vi "autorampturn.vi"() -> ()   [LabVIEW 2012, in "MainProject.lvrbt"]
uses:
  MainProject.lvrbt
  <vilib>/NXT/Hardware/Plugins/Tetrix DC Motor/TetrixDCMotorAddress.ctl
  Drivers/AutoDriverControl.ctl
  FTC 2012 - 2013/Controls/SpeedControl.ctl
  <vilib>/NXT/HiTechnic/HiTechnic Controls/HiTechnic Port.ctl
  <vilib>/NXT/Block Support/NXT_InputPort.ctl
  <vilib>/NXT/NXTIO Xnodes/NXTIONodeSubVIs/TETRIX IO Check Battery.vi
  <vilib>/NXT/Dual Mode Library/Waits/Wait_Num(msec).vi
  <vilib>/NXT/NXTIO Xnodes/NXTIONodeSubVIs/TETRIX IO Stop DC Motors.vi
  <vilib>/NXT/Subs/LVHSConnector.ctl
  <vilib>/NXT/NXTIO Xnodes/AddressXNode/NXTIOAddress.xnode
  BlankTemplates/BlankTemplates.lvrbt
  <vilib>/NXT/NXTIO Xnodes/NXTIOXNode/NXTIO.xnode
  <vilib>/NXT/LegoClasses/BrickReference/BrickReference.lvclass
panel:
  out "Enabled":bool
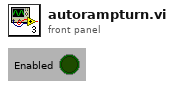
[diagram p1: front panel]
types:
  T1 = typedef "LVHSConnector.ctl" = refnum<class "BrickReference.lvclass">
  T2 = typedef "TetrixDCMotorAddress.ctl" = i16
  T3 = typedef "SpeedControl.ctl" = enum16{"Fast", "Medium", "Slow"}
  T4 = typedef "AutoDriverControl.ctl" = enum16{"Init", "Forward", "Reverse", "Left", "Right", "Brake"}
  T5 = typedef "HiTechnic Port.ctl" = cluster{"Port":T6, "MUX Port":u8}
  T6 = typedef "NXT_InputPort.ctl" = u8
  T7 = cluster{"TetrixDCMotor":T2, "TetrixDCMotor 2":T2}
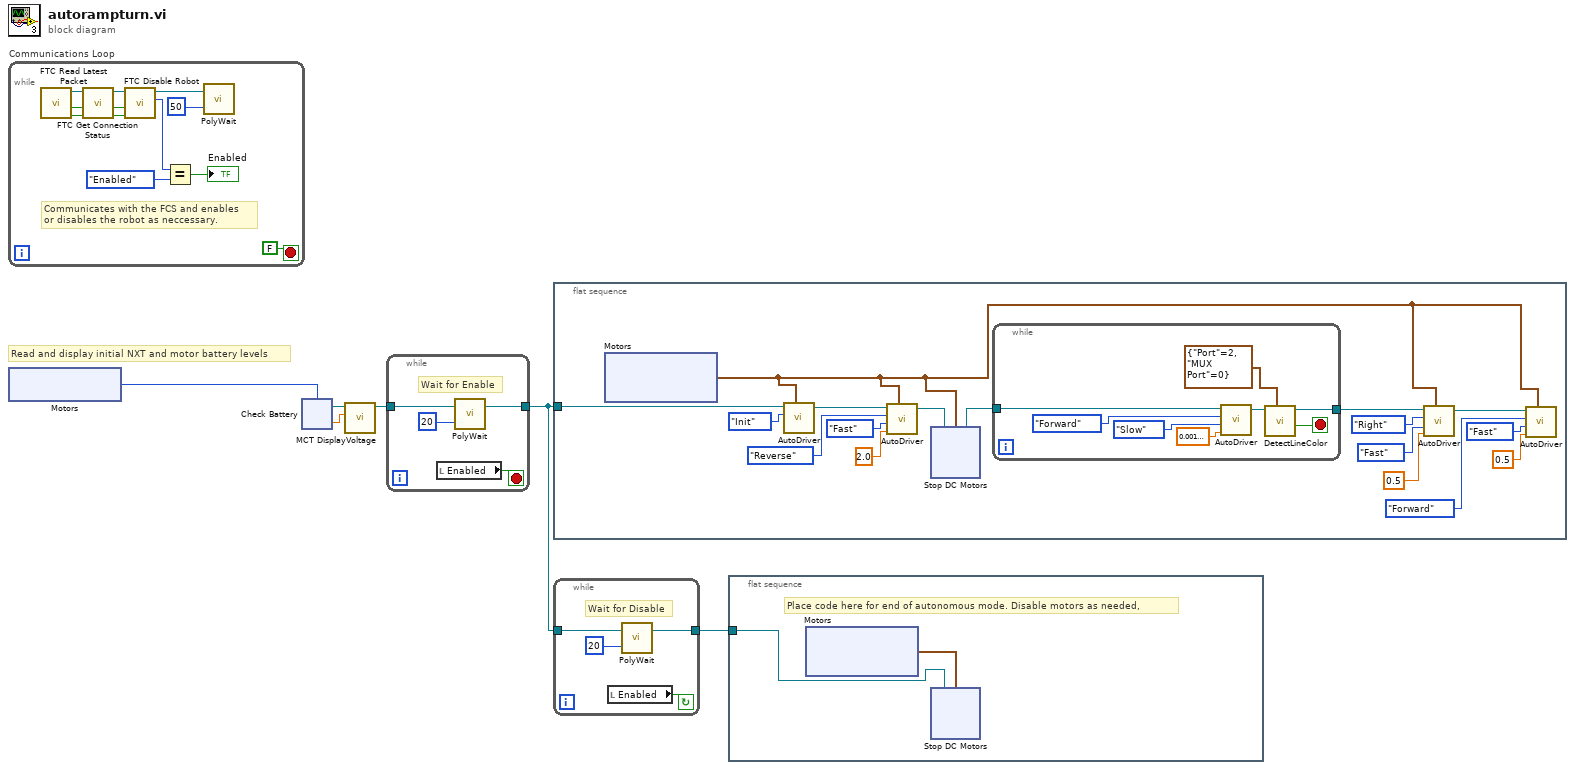
[diagram p0: block diagram]
diagram:
  # "Read and display initial NXT and motor battery levels"
  n1 = while "Communications Loop" {
    stop <- FALSE stop-if-true
    # "Communicates with the FCS and enables \nor disables the robot as neccessary."
    n2 = call <vilib>:"FTC Read Latest Packet.vi"() -> ("Packet Received?"=w16:bool, "Stopped?"=w15:bool, "NXT"=w18:T1)  [unwired: 6 in, 3 out]
    n3 = call <vilib>:"FTC Get Connection Status.vi"("Packet Received?"=w16, "Stopped?"=w15, "NXT"=w18) -> ("Online?"=w7:bool, "Stopped?"=w8:bool, "NXT"=w17:T1)  [unwired: 5 in]
    n4 = call <vilib>:"FTC Disable Robot.vi"("Online?"=w7, "Stopped?"=w8, "NXT"=w17) -> ("Enabled?"=w11:enum16{"Disabled", "Enabled"}, "NXT"=w13:T1)  [unwired: 3 in]
    n5 = Equal?(x=w11, y=enum16{"Disabled", "Enabled"}."Enabled") -> (x = y?=→"Enabled":bool)
    n6 = call-poly <vilib>:"PolyWait.vi"("Time (100 msec)"=u32 50 ("Time (msec)"), "NXT"=w13) -> ()  [unwired: 2 in, 1 out]
  }
  n7 = xnode "Motors"() -> ("Motor"=w6:T2)
  n8 = xnode "Check Battery"("Motors"=w6) -> ("Voltage 1"=w1:sgl, "NXT"=w3:T1)  [unwired: 1 in]
  n9 = call <vilib>:"MCT DisplayVoltage.vi"("Motor Voltage"=w1, "NXT"=w3) -> ("NXT"=w2:T1)  [unwired: 9 in]
  n10 = while {
    tunnel: [w20] -> w5
    tunnel: w2 -> [w19]
    stop <- w21 stop-if-true
    # "Wait for Enable"
    n11 = local read "Enabled"() -> (w21:bool)
    n12 = call-poly <vilib>:"PolyWait.vi"("Time (100 msec)"=u32 20 ("Time (msec)"), "NXT"=w19) -> ("NXT"=w20:T1)  [unwired: 2 in]
  }
  n13 = flat-sequence {
    tunnel: w5 -> [w39]
    frame #0 {
      n14 = xnode "Motors"() -> ("Motor"=w24:cluster{"TetrixDCMotor":T2, "TetrixDCMotor":T2})
      n15 = call "AutoDriver.vi"("NXT In"=w39, "Motors"=w24, "Direction"=AutoDriverControl."Init") -> ("NXT Out"=w37:T1)  [unwired: 5 in]
      n16 = call "AutoDriver.vi"("NXT In"=w37, "Motors"=w24, "Direction"=AutoDriverControl."Reverse", "Speed"=SpeedControl."Fast", "Time (1 sec)"=sgl 2.0) -> ("NXT Out"=w33:T1)  [unwired: 3 in]
      n17 = xnode "Stop DC Motors"("Motors"=w24, "NXT"=w33) -> ("NXT"=w32:T1)
      n18 = while {
        tunnel: w32 -> [w47]
        tunnel: [w45] -> w23
        stop <- w40 stop-if-true
        n19 = call "AutoDriver.vi"("NXT In"=w47, "Direction"=AutoDriverControl."Forward", "Speed"=SpeedControl."Slow", "Time (1 sec)"=sgl 0.001) -> ("NXT Out"=w44:T1)  [unwired: 4 in]
        n20 = call "DetectLineColor.vi"("Port/MUX"=T5 {"Port"=2, "MUX Port"=0}, "NXT In"=w44) -> ("Detected Line?"=w40:bool, "NXT Out"=w45:T1)  [unwired: 7 in, 1 out]
      }
      n21 = call "AutoDriver.vi"("NXT In"=w23, "Motors"=w24, "Direction"=AutoDriverControl."Right", "Speed"=SpeedControl."Fast", "Time (1 sec)"=sgl 0.5) -> ("NXT Out"=w25:T1)  [unwired: 3 in]
      n22 = call "AutoDriver.vi"("NXT In"=w25, "Motors"=w24, "Direction"=AutoDriverControl."Forward", "Speed"=SpeedControl."Fast", "Time (1 sec)"=sgl 0.5) -> ()  [unwired: 3 in, 1 out]
    }
  }
  n23 = while {
    tunnel: [w57] -> w4
    tunnel: w5 -> [w56]
    stop <- w58 continue-if-true
    # "Wait for Disable"
    n24 = local read "Enabled"() -> (w58:bool)
    n25 = call-poly <vilib>:"PolyWait.vi"("Time (100 msec)"=u32 20 ("Time (msec)"), "NXT"=w56) -> ("NXT"=w57:T1)  [unwired: 2 in]
  }
  n26 = flat-sequence {
    tunnel: w4 -> [w61]
    frame #0 {
      # "Place code here for end of autonomous mode. Disable motors as needed,"
      n27 = xnode "Motors"() -> ("Motor"=w60:cluster{"TetrixDCMotor":T2, "TetrixDCMotor":T2})
      n28 = xnode "Stop DC Motors"("Motors"=w60, "NXT"=w61) -> ()  [unwired: 1 out]
    }
  }
